vi "Connect.vi"(8 "error in":errorcluster, 11 "6509 in":refnum<class "6509.lvclass">) -> (0 "error out":errorcluster, 3 "6509 out":refnum<class "6509.lvclass">)   [LabVIEW 2019, in "6509.lvlib" / "6509.lvclass"]
uses:
  Library/6509.lvclass
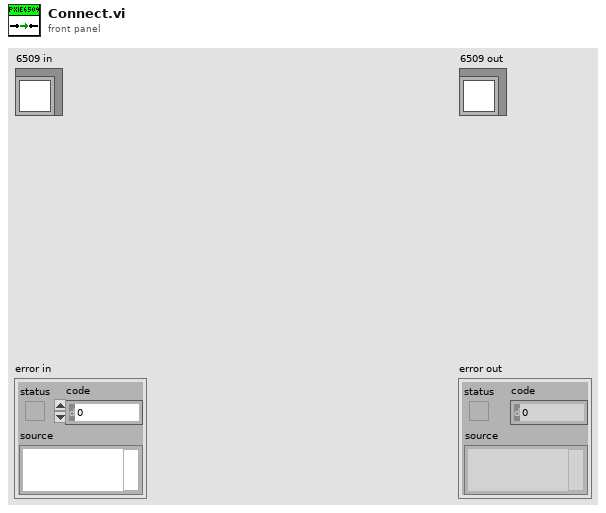
[diagram p1: front panel]
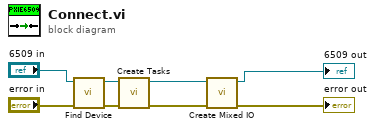
[diagram p0: block diagram]
diagram:
  n1 = call "Find Device.vi"("error in"="error in", "6509 in"="6509 in") -> ("error out"=w4:errorcluster, "6509 out"=w3:refnum<class "6509.lvclass">)  [unwired: 8 in]
  n2 = call "Create Tasks.vi"("error in"=w4, "6509 in"=w3) -> ("error out"=w8:errorcluster, "6509 out"=w7:refnum<class "6509.lvclass">)  [unwired: 8 in]
  n3 = call "Create Mixed IO.vi"("error in"=w8, "6509 in"=w7) -> ("error out"=→"error out":errorcluster, "6509 out"=→"6509 out":refnum<class "6509.lvclass">)  [unwired: 8 in]
